vi "LvVariantsFromString.vi"(8 "error IO":errorcluster, 11 "iniString":string="[SIAM_test_Standalone]\n<LvVariant>\n<Name>Variant Data</Name>\n<String>\n<Name>address</Name>\n<Val>192.168.1.160</Val>\n</String>\n</LvVariant>\n\n<LvVariant>\n<Name>Variant Data</Name>\n<String>\n<Name>instrument name</Name>\n<Val>xavier32-2</Val>\n</String>\n</LvVariant>\n\n<LvVariant>\n<Name>Variant Data</Name>\n<Cluster>\n<Name>Axis</Name>\n<NumElts>15</NumElts>\n<Cluster>\n<Name>Linear</Name>\n<NumElts>2</NumElts>\n<U32>\n<Name>Axis-Ring</Name>\n<Val>16777217</Val>\n</U32>\n<I32>\n<Name>Position</Name>\n<Val>1021459</Val>\n</I32>\n</Cluster>\n<Cluster>\n<Name>Linear</Name>\n<NumElts>2</NumElts>\n<U32>\n<Name>Axis-Ring</Name>\n<Val>17825793</Val>\n</U32>\n<I32>\n<Name>Position</Name>\n<Val>463519</Val>\n</I32>\n</Cluster>\n<Cluster>\n<Name>Linear 2</Name>\n<NumElts>2</NumElts>\n<U32>\n<Name>Axis-Ring</Name>\n<Val>104857665</Val>\n</U32>\n<I32>\n<Name>Position</Name>\n<Val>689614</Val>\n</I32>\n</Cluster>\n<Cluster>\n<Name>Linear 3</Name>\n<NumElts>2</NumElts>\n<U32>\n<Name>Axis-Ring</Name>\n<Val>20971521</Val>\n</U32>\n<I32>\n<Name>Position</Name>\n<Val>0</Val>\n</I32>\n</Cluster>\n<Cluster>\n<Name>Linear</Name>\n<NumElts>2</NumElts>\n<U32>\n<Name>Axis-Ring</Name>\n<Val>22020097</Val>\n</U32>\n<I32>\n<Name>Position</Name>\n<Val>0</Val>\n</I32>\n</Cluster>\n<Cluster>\n<Name>Linear 4</Name>\n<NumElts>2</NumElts>\n<U32>\n<Name>Axis-Ring</Name>\n<Val>2684354561</Val>\n</U32>\n<I32>\n<Name>Position</Name>\n<Val>0</Val>\n</I32>\n</Cluster>\n<Cluster>\n<Name>Linear 5</Name>\n<NumElts>2</NumElts>\n<U32>\n<Name>Axis-Ring</Name>\n<Val>2685403137</Val>\n</U32>\n<I32>\n<Name>Position</Name>\n<Val>0</Val>\n</I32>\n</Cluster>\n<Cluster>\n<Name>Linear 6</Name>\n<NumElts>2</NumElts>\n<U32>\n<Name>Axis-Ring</Name>\n<Val>2687500289</Val>\n</U32>\n<I32>\n<Name>Position</Name>\n<Val>0</Val>\n</I32>\n</Cluster>\n<Cluster>\n<Name>Linear 7</Name>\n<NumElts>2</NumElts>\n<U32>\n<Name>Axis-Ring</Name>\n<Val>2691694593</Val>\n</U32>\n<I32>\n<Name>Position</Name>\n<Val>0</Val>\n</I32>\n</Cluster>\n<Cluster>\n<Name>Linear 8</Name>\n<NumElts>2</NumElts>\n<U32>\n<Name>Axis-Ring</Name>\n<Val>2701131777</Val>\n</U32>\n<I32>\n<Name>Position</Name>\n<Val>0</Val>\n</I32>\n</Cluster>\n<Cluster>\n<Name>Linear 9</Name>\n<NumElts>2</NumElts>\n<U32>\n<Name>Axis-Ring</Name>\n<Val>2717908993</Val>\n</U32>\n<I32>\n<Name>Position</Name>\n<Val>0</Val>\n</I32>\n</Cluster>\n<Cluster>\n<Name>Linear 10</Name>\n<NumElts>2</NumElts>\n<U32>\n<Name>Axis-Ring</Name>\n<Val>2718957569</Val>\n</U32>\n<I32>\n<Name>Position</Name>\n<Val>0</Val>\n</I32>\n</Cluster>\n<Cluster>\n<Name>Linear 11</Name>\n<NumElts>2</NumElts>\n<U32>\n<Name>Axis-Ring</Name>\n<Val>2720006145</Val>\n</U32>\n<I32>\n<Name>Position</Name>\n<Val>0</Val>\n</I32>\n</Cluster>\n<Cluster>\n<Name>Linear 12</Name>\n<NumElts>2</NumElts>\n<U32>\n<Name>Axis-Ring</Name>\n<Val>2721054721</Val>\n</U32>\n<I32>\n<Name>Position</Name>\n<Val>0</Val>\n</I32>\n</Cluster>\n<Cluster>\n<Name>Linear 13</Name>\n<NumElts>2</NumElts>\n<U32>\n<Name>Axis-Ring</Name>\n<Val>67108865</Val>\n</U32>\n<I32>\n<Name>Position</Name>\n<Val>150000</Val>\n</I32>\n</Cluster>\n</Cluster>\n</LvVariant>\n\n<LvVariant>\n<Name>Variant Data</Name>\n<Cluster>\n<Name>User</Name>\n<NumElts>4</NumElts>\n<I32>\n<Name>z-distance_motorunits</Name>\n<Val>100</Val>\n</I32>\n<U16>\n<Name>#planes</Name>\n<Val>1</Val>\n</U16>\n<EB>\n<Name>Digital-out</Name>\n<Val>22</Val>\n</EB>\n<U16>\n<Name>NoOfPhaseImages</Name>\n<Val>7</Val>\n</U16>\n</Cluster>\n</LvVariant>\n\n<LvVariant>\n<Name>Variant Data</Name>\n<Cluster>\n<Name>Constants</Name>\n<NumElts>17</NumElts>\n<I16>\n<Name>galvox-Line0</Name>\n<Val>5480</Val>\n</I16>\n<DBL>\n<Name>GalvoX-Blanking</Name>\n<Val>5500.0</Val>\n</DBL>\n<DBL>\n<Name>galvox-count/pix</Name>\n<Val>-2.4470</Val>\n</DBL>\n<I32>\n<Name>Camera-StartLine</Name>\n<Val>-62</Val>\n</I32>\n<U32>\n<Name>Camera-Endline</Name>\n<Val>3500</Val>\n</U32>\n<DBL>\n<Name>Wobbel-total</Name>\n<Val>4055.0</Val>\n</DBL>\n<U32>\n<Name>SM_ticks</Name>\n<Val>20</Val>\n</U32>\n<U32>\n<Name>Trigger_ticks</Name>\n<Val>100</Val>\n</U32>\n<DBL>\n<Name>galvoxAccel</Name>\n<Val>5.00000000000000</Val>\n</DBL>\n<DBL>\n<Name>WobbelAccel</Name>\n<Val>1.00000000000000E-2</Val>\n</DBL>\n<DBL>\n<Name>zAccel</Name>\n<Val>5.00000000000000E-2</Val>\n</DBL>\n<U32>\n<Name>z-delay-ticks</Name>\n<Val>700</Val>\n</U32>\n<DBL>\n<Name>SCMOS-LineSpeed [10µs]</Name>\n<Val>1.33889</Val>\n</DBL>\n<U16>\n<Name>RS height- Pix</Name>\n<Val>80</Val>\n</U16>\n<DBL>\n<Name>extra-xgalvo</Name>\n<Val>78.0</Val>\n</DBL>\n<U32>\n<Name>zcommand</Name>\n<Val>4026531840</Val>\n</U32>\n<DBL>\n<Name>min turn ticks</Name>\n<Val>500.00000000000000</Val>\n</DBL>\n</Cluster>\n</LvVariant>\n\n<LvVariant>\n<Name>Variant Data</Name>\n<U8>\n<Name>UART=0..3</Name>\n<Val>2</Val>\n</U8>\n</LvVariant>\n\n<LvVariant>\n<Name>Variant Data</Name>\n<Cluster>\n<Name>TSM</Name>\n<NumElts>4</NumElts>\n<U8>\n<Name>RS232-axis</Name>\n<Val>255</Val>\n</U8>\n<U8>\n<Name>axis</Name>\n<Val>255</Val>\n</U8>\n<String>\n<Name>Command</Name>\n<Val>?TILL_STATUS</Val>\n</String>\n<DBL>\n<Name>value</Name>\n<Val>946.00000000000000</Val>\n</DBL>\n</Cluster>\n</LvVariant>\n\n<LvVariant>\n<Name>Variant Data</Name>\n<String>\n<Name>String</Name>\n<Val>SOUR2=POW:LEV:IMM:AMPL?\n\n</Val>\n</String>\n</LvVariant>\n") -> (0 "error out":errorcluster, 3 "Array":cluster{"LvVariant":string, "Name":string}[](array[cluster]))   [LabVIEW 2011]
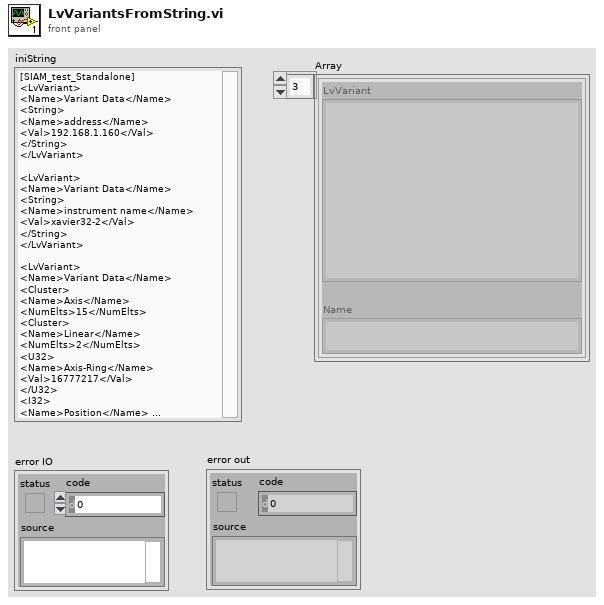
[diagram p1: front panel]
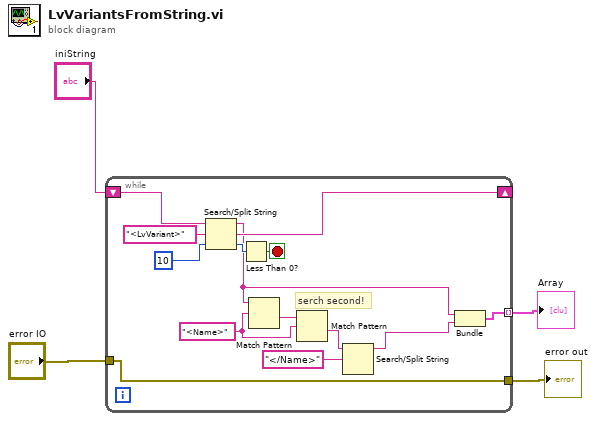
[diagram p0: block diagram]
diagram:
  n1 = while {
    tunnel: "error IO" -> [w5]
    shift-right: [w13] -> _
    shift-left: "iniString" -> [w14]
    tunnel: [w6] -> w2 mode=indexing
    tunnel: [w5] -> w1
    stop <- w9 stop-if-true
    w17 = "<Name>" ("saerch")
    # "serch second!"
    n2 = Search/Split String(string=w14, search string/char (-)="<LvVariant>", offset (0)=10) -> (substring before match=w8:string, match + rest of string=w13:string, offset of match=w10:i32)
    n3 = Less Than 0?(x=w10) -> (x < 0?=w9:bool)
    n4 = Match Pattern(string=w8, regular expression=w17) -> (after substring=w16:string)  [unwired: 1 in, 3 out]
    n5 = Match Pattern(string=w16, regular expression=w17) -> (after substring=w15:string)  [unwired: 1 in, 3 out]
    n6 = Search/Split String(string=w15, search string/char (-)="</Name>") -> (substring before match=w7:string)  [unwired: 1 in, 2 out]
    n7 = Bundle("iniString"=w8, "iniString"=w7) -> (w6:cluster{"iniString":string, "iniString":string})  [unwired: 1 in]
  }
  "Array" <- w2
  "error out" <- w1
